vi "Feeder Disponible Global.vi"() -> ()   [LabVIEW 2015]
panel:
  in  "Can feed":bool
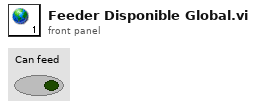
[diagram p1: front panel]
diagram:
